vi "Actor Core.vi"(8 "error in":errorcluster, 11 "Graph in":refnum<class "Graph.lvclass">) -> (0 "error out":errorcluster, 3 "Actor out":refnum<class "Actor.lvclass">)   [LabVIEW 2020, in "Graph.lvlib" / "Graph.lvclass"]
doc: "(<B>Filename</B>: Actor Framework.lvlib:Actor.lvclass:Actor Core.vi)\n\nReceives messages to the actor, reacts to them, and initiates any error handling that may shut the actor down.\n\nDescendant classes may override this VI to append parallel tasks for the actor to complete while it handles messages. Overrides use the Call Parent Method node.\n\nThis implementation plot Data in a chart using the To Waveform method of the Data class."
uses:
  Graph.lvclass
  C:/Current projects/WS/PPL/HDH.Actor Framework.Core.Actor.lvlibp/1abvi3w/vi.lib/ActorFramework/Actor/Actor.lvclass
  PPL/HDH.Actor Framework.Core.Actor.lvlibp/1abvi3w/vi.lib/ActorFramework/Actor/Actor.lvclass
  Graph.lvclass/Graph.ctl
  PPL/HDH.Data.Generic.lvlibp/Data.lvclass
  PPL/HDH.Actor Framework.Core.Actor.lvlibp/1abvi3w/vi.lib/ActorFramework/Stop Msg/Stop Msg.lvclass
panel:
  out "Waveform Chart":waveform(dbl)[](graph)
  in  "Pause":bool
  in  "Clear":bool
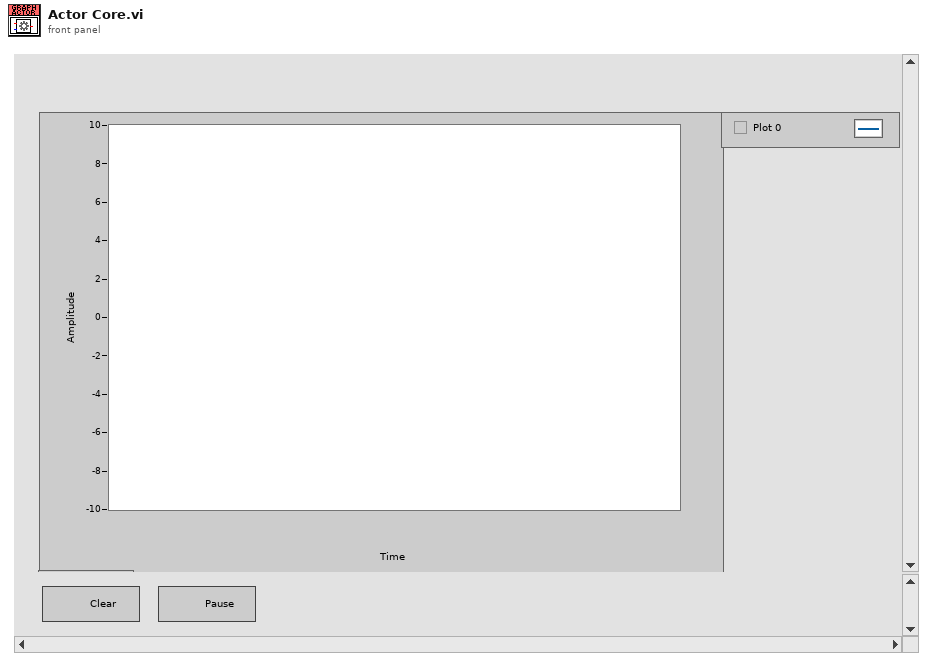
[diagram p1: front panel]
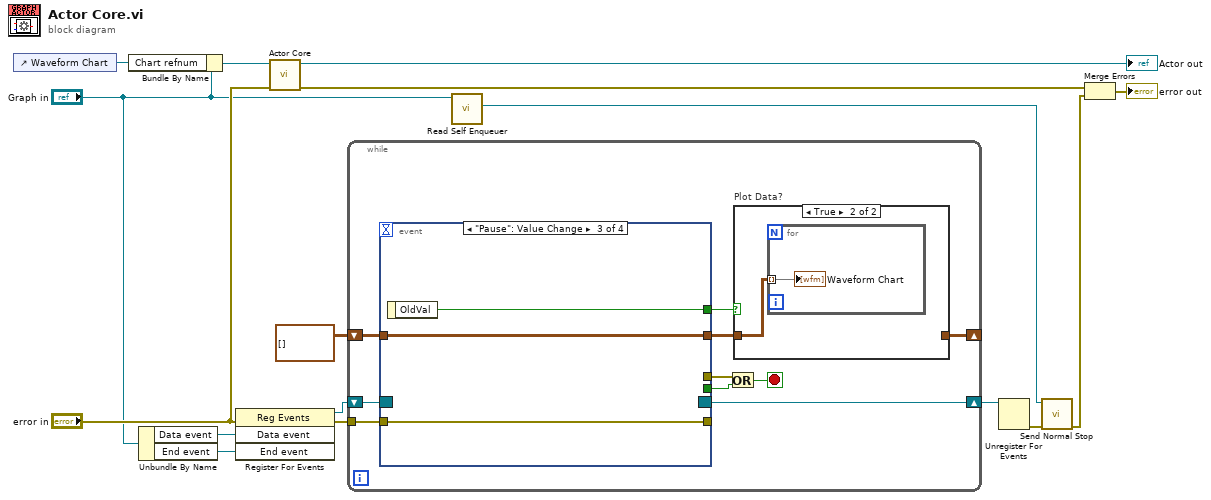
[diagram p0: block diagram]
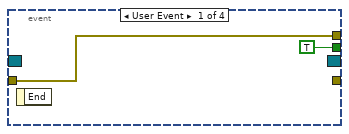
[diagram p3: hidden frame]
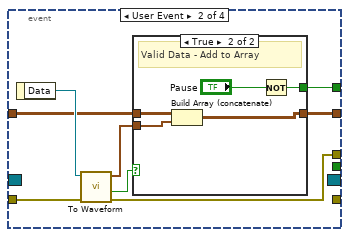
[diagram p4: hidden frame]
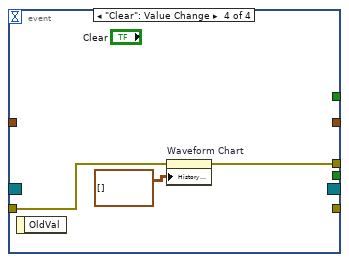
[diagram p6: hidden frame]
diagram:
  n1 = control-ref of="Waveform Chart"() -> (w13:refnum<vi>)
  n2 = Bundle By Name(cluster="Graph in", "Chart refnum"=w13) -> (w14:refnum<class "Graph.lvclass">)
  n3 = Unbundle By Name("Graph in") -> ("Data event"=w12:refnum<user-event>, "End event"=w11:refnum<user-event>)
  n4 = register-events(error in="error in", w12, w11) -> (reference out=w10:refnum<event-registration>, error out=w7:errorcluster)  [unwired: 1 in]
  n5 = call-parent "Actor Core.vi"("error in"="error in", "Actor in"=w14) -> ("error out"=w16:errorcluster, "Actor out"=→"Actor out":refnum<class "Actor.lvclass">)  [unwired: 8 in]
  n6 = while {
    shift-right: [w25] -> w9
    shift-left: w10 -> [w26]
    tunnel: w7 -> [w23]
    shift-right: [w17] -> _
    shift-left: waveform(dbl)[][] [] ("Waveform Array") -> [w20]
    stop <- w22 stop-if-true
    n7 = event shown="[2] \"Pause\": Value Change" {
      selector: w26 -> [_ _ _ _]
      dyn-events: [_ _ _ _] -> w25
      timeout: _ -> [_ _ _ _]
      tunnel: [TRUE _ _ _] -> w24
      tunnel: w23 -> [w30 w37 w47 w51]
      tunnel: [w30 w36 _ w50] -> w21
      tunnel: [_ w32 w46 _] -> w18
      tunnel: w20 -> [_ w34 w46 _]
      tunnel: [_ w33 w48 _] -> w19
      tunnel: [_ _ w47 _] -> _
      event User Event {
        n8 = event-data() -> ()  [unwired: 1 in, 1 out]
      }
      event User Event {
        n9 = event-data() -> ("Data"=w39:refnum<class "Data.lvclass">)  [unwired: 1 in]
        n10 = call-dynamic "To Waveform.vi"("error in (no error)"=w37, "Data in"=w39) -> ("error out"=w36:errorcluster, "Success?"=w35:bool, "Waveform Array"=w38:waveform(dbl)[])  [unwired: 7 in]
        n11 = case shown="True" w35 {
          tunnel: w38 -> [_ w44]
          tunnel: w34 -> [w40 w45]
          tunnel: [w40 w43] -> w32
          tunnel: [_ w41] -> w33
          frame False {
            # "Invalid Data - Drop Data"
          }
          frame True {
            # "Valid Data - Add to Array"
            n12 = Build Array (concatenate)(w45, w44) -> (w43:waveform(dbl)[][])
            n13 = Not(x="Pause") -> (.not. x?=w41:bool)
          }
        }
      }
      event "Pause": Value Change {
        n14 = event-data() -> ("OldVal"=w48:bool)  [unwired: 1 in]
      }
      event "Clear": Value Change {
        n15 = event-data() -> ()  [unwired: 1 in, 1 out]
        n16 = property on="Waveform Chart" class="WFChart (strict)"(error in=w51, "History Data"=waveform(dbl)[][] []) -> (error out=w50:errorcluster)  [unwired: 1 in, 1 out]
      }
    }
    n17 = Or(x=w21, y=w24) -> (x .or. y?=w22:bool)
    n18 = case "Plot Data?" shown="True" w19 {
      tunnel: w18 -> [w27 w28]
      tunnel: [w27 _] -> w17
      frame False {
      }
      frame True {
        n19 = for {
          tunnel: w28 -> [w29] mode=indexing
          "Waveform Chart" <- w29
        }
      }
    }
  }
  n20 = call "Read Self Enqueuer.vi"("Actor"="Graph in") -> ("Self Enqueuer"=w4:refnum<class "Message Enqueuer.lvclass">)  [unwired: 10 in]
  n21 = Unregister For Events(event registration refnum=w9) -> (error out=w5:errorcluster)  [unwired: 1 in]
  n22 = call "Send Normal Stop.vi"("error in (no error)"=w5, "Message Enqueuer"=w4) -> ("error out"=w2:errorcluster)  [unwired: 9 in]
  n23 = Merge Errors(w16, w2) -> (→"error out":errorcluster)
